vi "Proj.vi"(0 "th_max":dbl, 1 "a":dbl, 2 "th":dbl, 3 "th_min":dbl, 4 "error in (no error)":errorcluster) -> (5 "Proj_th (a)":dbl, 6 "error out":errorcluster)   [LabVIEW 2021]
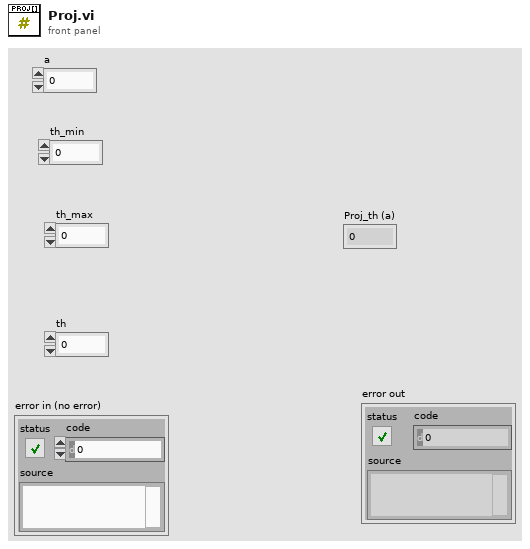
[diagram p1: front panel]
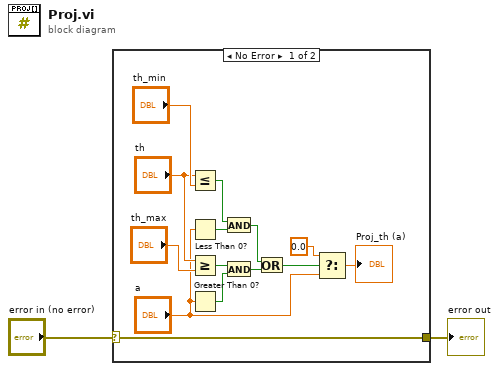
[diagram p0: block diagram]
diagram:
  n1 = case shown="No Error" "error in (no error)" {
    selector: "error in (no error)" -> [w16 w17]
    tunnel: [w16 w17] -> w1
    frame No Error {
      n2 = Less Or Equal?(x="th", y="th_min") -> (x <= y?=w12:bool)
      n3 = Less Than 0?(x="a") -> (x < 0?=w11:bool)
      n4 = Greater Or Equal?(x="th", y="th_max") -> (x >= y?=w6:bool)
      n5 = Greater Than 0?(x="a") -> (x > 0?=w4:bool)
      n6 = And(x=w12, y=w11) -> (x .and. y?=w9:bool)
      n7 = And(x=w6, y=w4) -> (x .and. y?=w3:bool)
      n8 = Or(x=w9, y=w3) -> (x .or. y?=w10:bool)
      n9 = Select(t=0.0, s=w10, f="a") -> (s? t:f=→"Proj_th (a)":dbl)
    }
    frame Error {
    }
  }
  "error out" <- w1
